vi "Run FGV Tests for 1D Double Array.vi"(2 "DELETE VI Reference":refnum<vi>, 3 "GET VI Reference":refnum<vi>, 4 "PUT VI Reference":refnum<vi>) -> (0 "Reason":string, 1 "Success":bool)   [LabVIEW 2013]
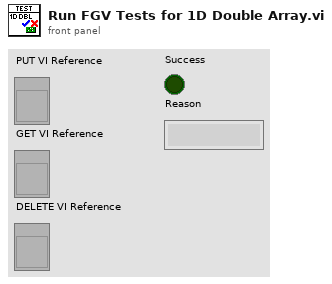
[diagram p1: front panel]
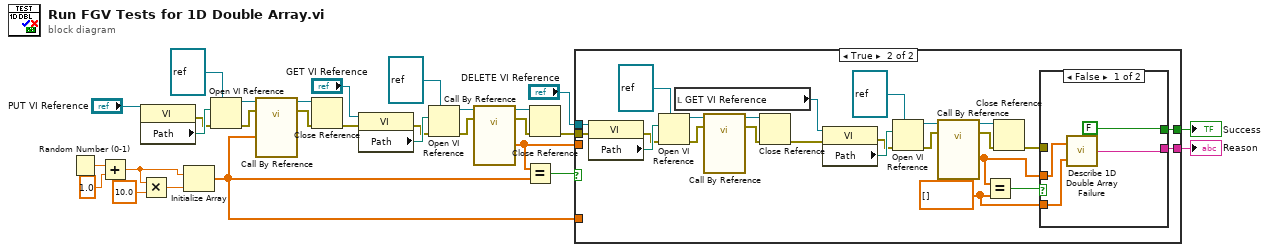
[diagram p0: block diagram]
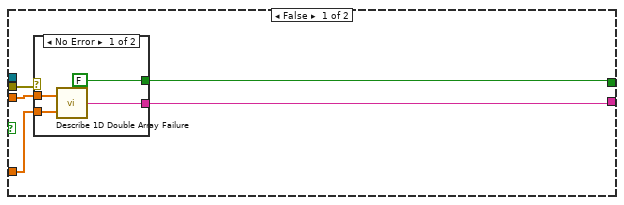
[diagram p2: hidden frame]
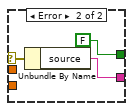
[diagram p3: hidden frame]
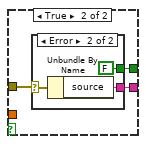
[diagram p4: hidden frame]
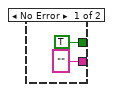
[diagram p5: hidden frame]
diagram:
  n1 = Random Number (0-1)() -> (number: 0 to 1=w14:dbl)
  n2 = Add(x=w14, y=1.0) -> (x+y=w2:dbl)
  n3 = property class="VI"(reference="PUT VI Reference") -> (error out=w7:errorcluster, "Path"=w20:path)  [unwired: 1 in, 1 out]
  n4 = Multiply(x=w2, y=10.0) -> (x*y=w3:dbl)
  n5 = Initialize Array(w2, w3) -> (w1:dbl[])
  n6 = Open VI Reference(type specifier VI Refnum (for type only)=refnum<vi> refnum, vi path=w20, error in (no error)=w7) -> (vi reference=w19:refnum<vi>, error out=w18:errorcluster)  [unwired: 3 in]
  n7 = call-by-ref "?"(reference=w19, error in=w18, "Force Data"=w1) -> (reference out=w17:refnum<vi>, error out=w16:errorcluster)
  n8 = Close Reference(reference=w17, error in (no error)=w16) -> (error out=w12:errorcluster)
  n9 = property class="VI"(reference="GET VI Reference", error in=w12) -> (error out=w8:errorcluster, "Path"=w25:path)  [unwired: 1 out]
  n10 = Open VI Reference(type specifier VI Refnum (for type only)=refnum<vi> refnum, vi path=w25, error in (no error)=w8) -> (vi reference=w26:refnum<vi>, error out=w27:errorcluster)  [unwired: 3 in]
  n11 = call-by-ref "?"(reference=w26, error in=w27) -> (reference out=w28:refnum<vi>, error out=w29:errorcluster, "Force Data"=w9:dbl[])
  n12 = Equal?(x=w9, y=w1) -> (x = y?=w10:bool)
  n13 = Close Reference(reference=w28, error in (no error)=w29) -> (error out=w11:errorcluster)
  n14 = case shown="True" w10 {
    tunnel: "DELETE VI Reference" -> [_ w59]
    tunnel: w11 -> [w30 w58]
    tunnel: w1 -> [w33 _]
    tunnel: w9 -> [w34 _]
    tunnel: [w32 w44] -> w6
    tunnel: [w31 w43] -> w5
    frame False {
      n15 = case shown="No Error" w30 {
        selector: w30 -> [_ w41]
        tunnel: w34 -> [w38 _]
        tunnel: w33 -> [w37 _]
        tunnel: [FALSE FALSE] -> w32
        tunnel: [w35 w39] -> w31
        frame No Error {
          n16 = call "Describe 1D Double Array Failure.vi"("Expected"=w37, "Got"=w38) -> ("Failure Description"=w35:string)
        }
        frame Error {
          n17 = Unbundle By Name(w41) -> ("source"=w39:string)
        }
      }
    }
    frame True {
      w42 = dbl[] [] ("initialized array")
      n18 = property class="VI"(reference=w59, error in=w58) -> (error out=w48:errorcluster, "Path"=w61:path)  [unwired: 1 out]
      n19 = Open VI Reference(type specifier VI Refnum (for type only)=refnum<vi> refnum, vi path=w61, error in (no error)=w48) -> (vi reference=w62:refnum<vi>, error out=w63:errorcluster)  [unwired: 3 in]
      n20 = local read "GET VI Reference"() -> (w46:refnum<vi>)
      n21 = call-by-ref "?"(reference=w62, error in=w63) -> (reference out=w64:refnum<vi>, error out=w65:errorcluster)  [unwired: 1 in]
      n22 = Close Reference(reference=w64, error in (no error)=w65) -> (error out=w51:errorcluster)
      n23 = property class="VI"(reference=w46, error in=w51) -> (error out=w49:errorcluster, "Path"=w53:path)  [unwired: 1 out]
      n24 = Open VI Reference(type specifier VI Refnum (for type only)=refnum<vi> refnum, vi path=w53, error in (no error)=w49) -> (vi reference=w54:refnum<vi>, error out=w55:errorcluster)  [unwired: 3 in]
      n25 = call-by-ref "?"(reference=w54, error in=w55) -> (reference out=w56:refnum<vi>, error out=w57:errorcluster, "Force Data"=w45:dbl[])
      n26 = Equal?(x=w45, y=w42) -> (x = y?=w50:bool)
      n27 = Close Reference(reference=w56, error in (no error)=w57) -> (error out=w47:errorcluster)
      n28 = case shown="False" w50 {
        tunnel: w47 -> [_ w72]
        tunnel: w45 -> [w69 _]
        tunnel: w42 -> [w68 _]
        tunnel: [FALSE w71] -> w44
        tunnel: [w66 w70] -> w43
        frame False {
          n29 = call "Describe 1D Double Array Failure.vi"("Expected"=w68, "Got"=w69) -> ("Failure Description"=w66:string)
        }
        frame True {
          n30 = case shown="Error" w72 {
            selector: w72 -> [_ w77]
            tunnel: [TRUE FALSE] -> w71
            tunnel: ["" ("source") w75] -> w70
            frame No Error {
            }
            frame Error {
              n31 = Unbundle By Name(w77) -> ("source"=w75:string)
            }
          }
        }
      }
    }
  }
  "Success" <- w6
  "Reason" <- w5
